vi "LabVIEW_Test_Detector_3.vi"() -> ()   [LabVIEW 2019]
uses:
  <vilib>/measure/madcrms.llb/Averaged DC-RMS for N Chan.vi
  <vilib>/measure/madcrms.llb/Basic Averaged DC-RMS for N Chan.vi
  <vilib>/measure/NI_MAPro.lvlib
panel:
  out "Waveform Graph":dynamicdata(graph)
  out "Photoplethismography Signal":waveform(dbl)[](graph)
  out "DC values":dbl[](array[numeric]) format="%.2p"
  in  "Record Data":bool
  out "Saving Data":bool
  in  "Filename":path=path "C:/Users/larry.theran.IRESS/Documents/Labview/New Data test/freq50p10.lvm"
  in  "?":bool
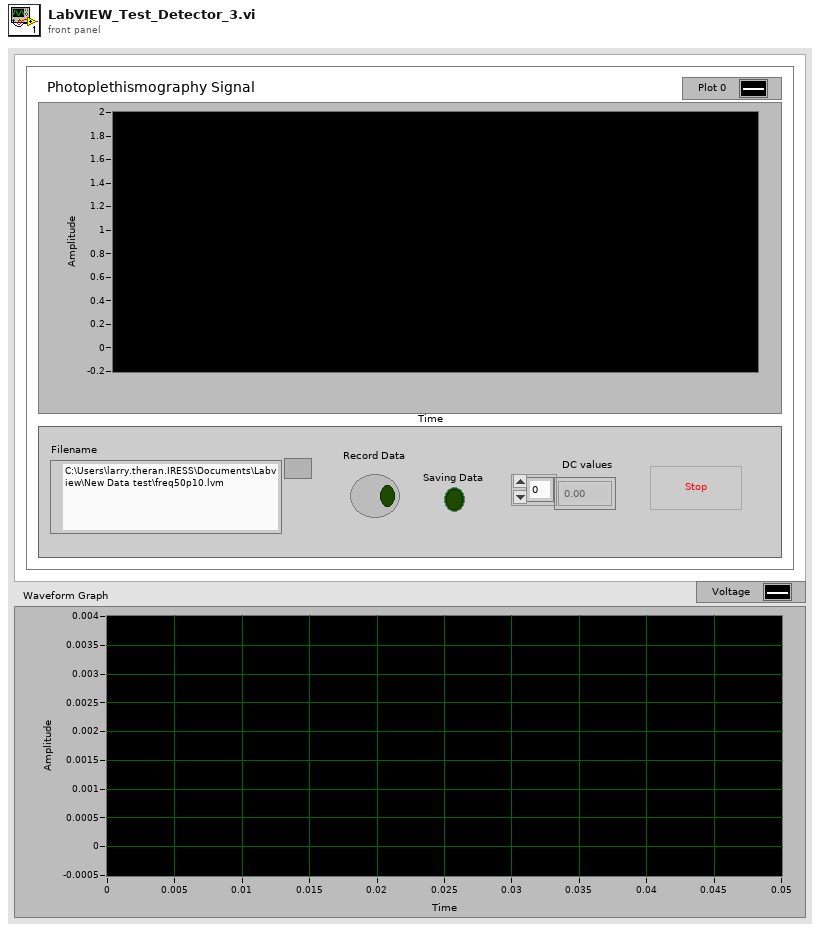
[diagram p1: front panel]
types:
  T1 = enum16{"Rectangular (none)", "Hanning", "Low side lobe"}
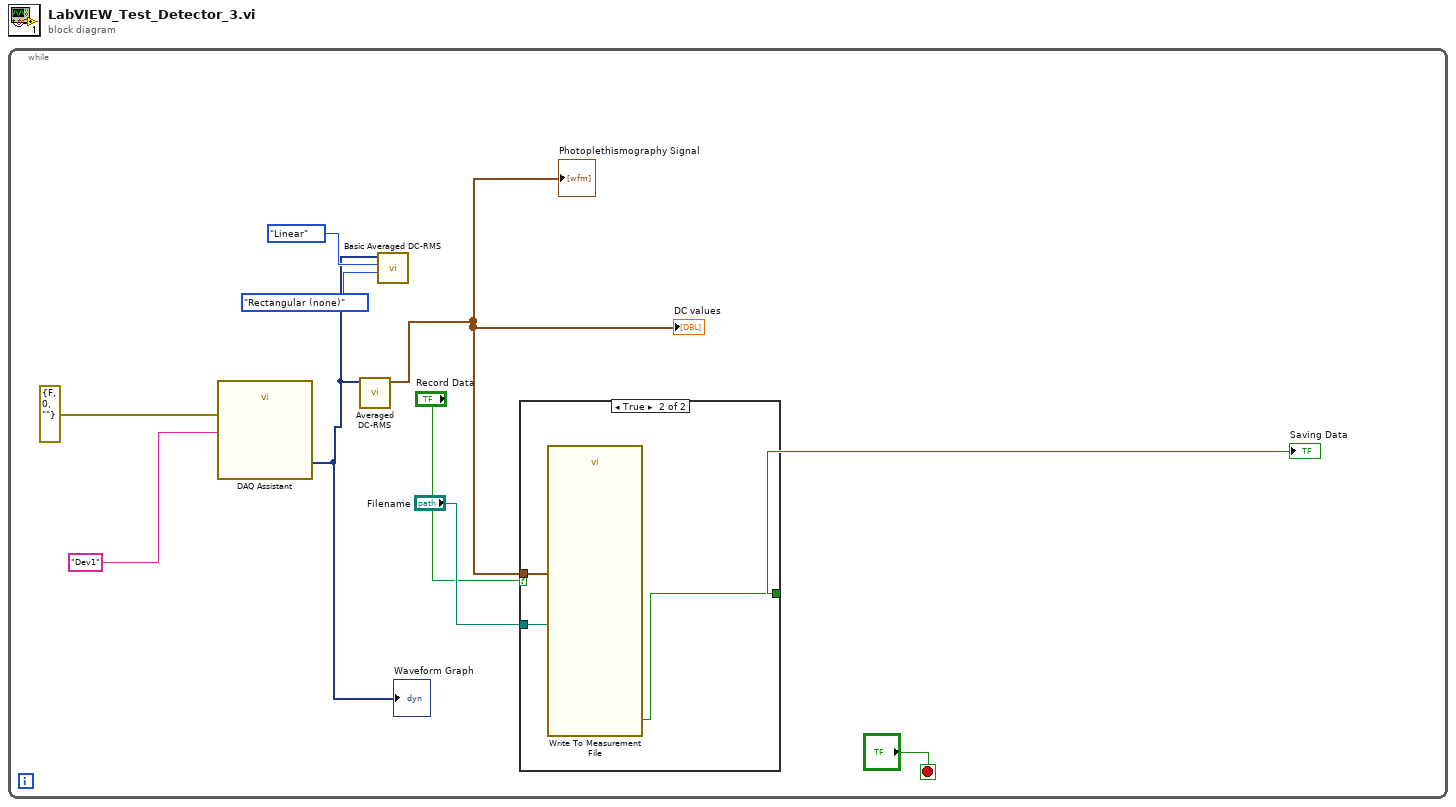
[diagram p0: block diagram]
diagram:
  n1 = while {
    stop <- "?" stop-if-true
    n2 = call "DAQ Assistant"("error in"=errorcluster {"status"=FALSE, "code"=0, "source"=""}, "device name"="Dev1") -> ("data"=w1:dynamicdata)  [unwired: 14 in, 3 out]
    "Waveform Graph" <- w1
    n3 = call-poly <vilib>:"Averaged DC-RMS.vi"("signals in"=w1) -> ("DC value waveforms"=w2:waveform(dbl)[])  [unwired: 6 in, 4 out]
    "DC values" <- w2
    "Photoplethismography Signal" <- w2
    n4 = call-poly <vilib>:"Basic Averaged DC-RMS.vi"("window"=T1."Rectangular (none)", "averaging type"=enum16{"Linear", "Exponential"}."Linear", "signals in"=w1) -> ()  [unwired: 5 in, 4 out]
    n5 = case shown="True" "Record Data" {
      tunnel: w2 -> [_ w13]
      tunnel: "Filename" -> [_ w12]
      tunnel: [_ w11] -> w6
      frame False {
      }
      frame True {
        n6 = call "Write To Measurement File"("Signals"=w13, "Filename"=w12) -> ("Saving Data"=w11:bool)  [unwired: 15 in, 2 out]
      }
    }
    "Saving Data" <- w6
  }
